vi "Ramping drive.vi"() -> ()   [LabVIEW 2017]
uses:
  <vilib>/Rock Robotics/WPI/ThirdParty/Phoenix-LabVIEW/Motor Controller/Controls/CTRE_Phoenix_MotorControl_ControlMode.ctl
  <vilib>/Rock Robotics/WPI/ThirdParty/Phoenix-LabVIEW/Motor Controller/Get/CTRE_Phoenix_MotorController_GetQuadratureData.vi
panel:
  in  "Max Speed/100Ms":dbl=650.0
  out "Acceleration Distance":dbl=8125.0
  in  "Ramp Seconds to full":dbl=2.5
  in  "Distance to Drive":dbl=5000.0
  in  "Distance tolerances":dbl=200.0
  out "TIMEOUTed":bool
  in  "TIMEOUT(S)":dbl=8.0
  # "NEED TALON DRIVE TO WORK"
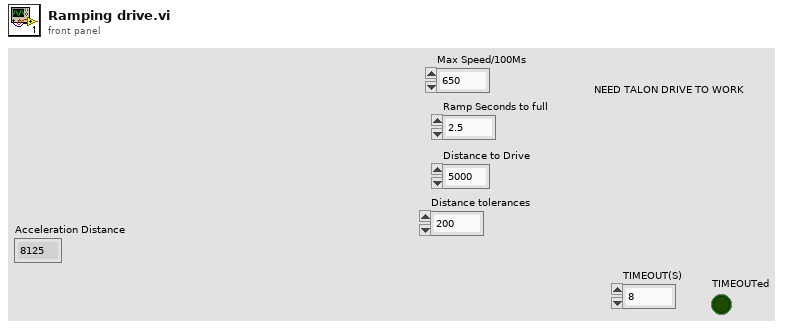
[diagram p1: front panel]
types:
  T1 = typedef "WPI_MotorControlDeviceRef.ctl" = cluster{"DeviceStatus":errorcluster, "Type":T2, "PWM":cluster{"PWM Channel":T3, "DeadBand":T4}, "CAN":cluster{"Device Number":u8, "SetOutput VI Ref":variant, "GetOutput VI Ref":variant, "Enable VI Ref":variant, "Disable VI Ref":variant, "Data":variant}, "Invert":bool, "DIO PWM":cluster{"PWM \"Enable\" Channel":T3, "DIOChannel":T5, "PWM Rate":dbl}}
  T2 = typedef "WPI_MotorControlType.ctl" = enum16{"PWM", "CAN", "DIO PWM"}
  T3 = typedef "FPGA_DIOPWMChannel.ctl" = enum8{"PWM 0", "PWM 1", "PWM 2", "PWM 3", "PWM 4", "PWM 5", "PWM 6", "PWM 7", "PWM 8", "PWM 9", "PWM MXP 0", "PWM MXP 1", "PWM MXP 2", "PWM MXP 3", "PWM MXP 4", "PWM MXP 5", "PWM MXP 6", "PWM MXP 7", "PWM MXP 8", "PWM MXP 9", "Invalid"}
  T4 = typedef "WPI_PWMDeadband.ctl" = cluster{"Name":string, "maxPositivePwm":i32, "minPositivePwm":i32, "centerPwm":i32, "maxNegativePwm":i32, "minNegativePwm":i32, "angularRange":u16}
  T5 = typedef "FPGA_DIOChannel.ctl" = enum8{"DIO 0", "DIO 1", "DIO 2", "DIO 3", "DIO 4", "DIO 5", "DIO 6", "DIO 7", "DIO 8", "DIO 9", "DIO MXP 0", "DIO MXP 1", "DIO MXP 2", "DIO MXP 3", "DIO MXP 4", "DIO MXP 5", "DIO MXP 6", "DIO MXP 7", "DIO MXP 8", "DIO MXP 9", "DIO MXP 10", "DIO MXP 11", "DIO MXP 12", "DIO MXP 13", "DIO MXP 14", "DIO MXP 15", "SPI Port CS1", "SPI Port CS2", "SPI Port CS3", "SPI Port MISO", "SPI Port MOSI", "Invalid"}
  T6 = typedef "CTRE_Phoenix_MotorControl_ControlMode.ctl" = u16
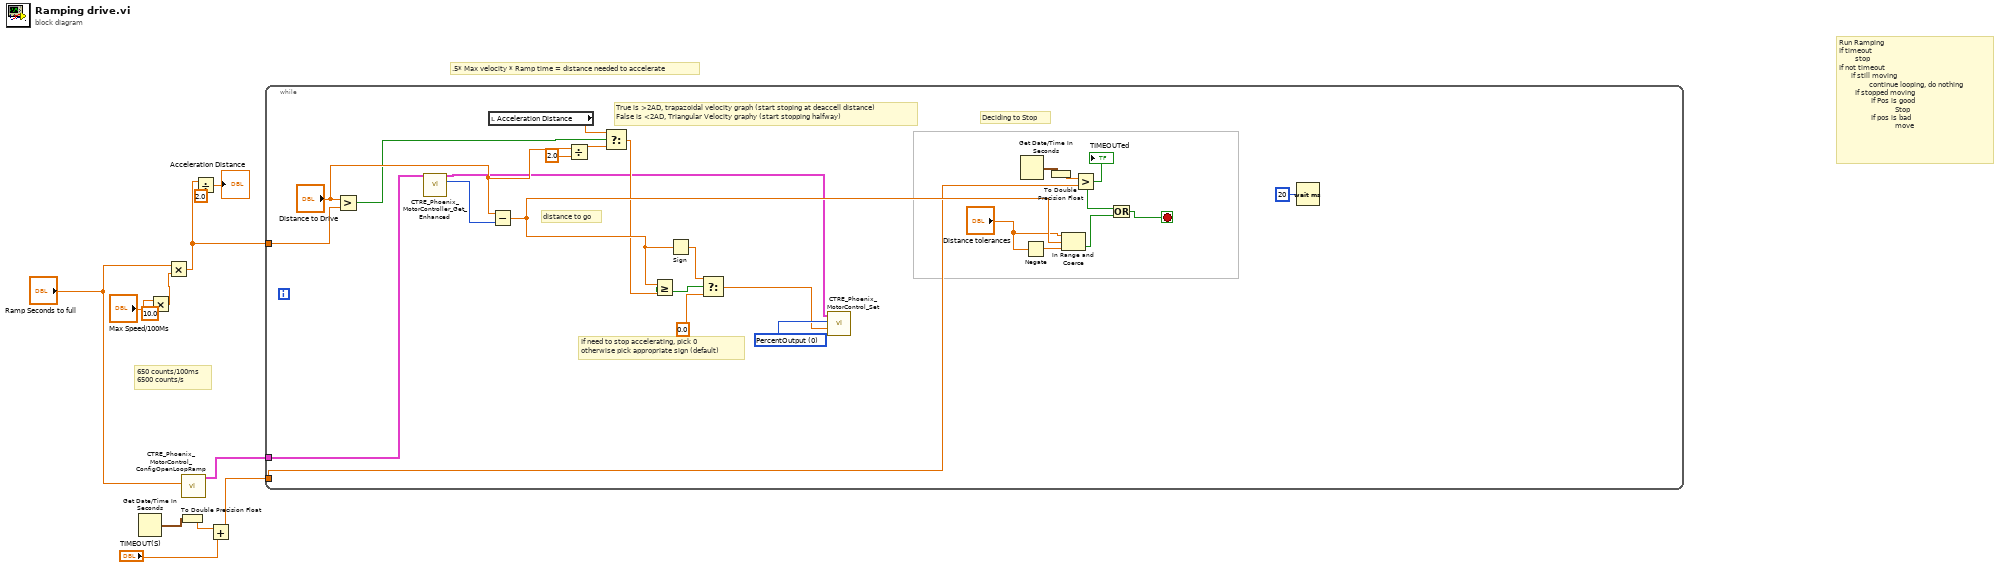
[diagram p0: block diagram]
diagram:
  # "Run Ramping\nIf timeout\n        stop\nIf not timeout\n      if still moving\n               continue looping, do nothing\n        If stopped moving\n                If Pos is good\n                            Stop\n                If pos is bad\n                            move"
  # ".5* Max velocity * Ramp time = distance needed to accelerate"
  # "650 counts/100ms\n6500 counts/s"
  n1 = Get Date/Time In Seconds() -> (seconds since 1Jan1904=w3:timestamp)
  n2 = Multiply(x="Max Speed/100Ms", y=10.0) -> (x*y=w6:dbl)
  n3 = Multiply(x="Ramp Seconds to full", y=w6) -> (x*y=w1:dbl)
  n4 = To Double Precision Float(number=w3) -> (double precision float=w2:dbl)
  n5 = call <vilib>:"CTRE_Phoenix_MotorControl_ConfigOpenLoopRamp.vi"("secondsFromNeutralToFull"="Ramp Seconds to full") -> (3:"PhoenixMotorControlDevRef"=w10:T1, 11:"PhoenixMotorControlDevRef"=w9:T1)  [unwired: 8 in, 1 out]
  n6 = Divide(x=w1, y=2.0) -> (x/y=→"Acceleration Distance":dbl)
  n7 = Add(x=w2, y="TIMEOUT(S)") -> (x+y=w4:dbl)
  n8 = while {
    tunnel: w10 -> [w39]
    tunnel: w4 -> [w36]
    tunnel: w1 -> [w34]
    stop <- w15 stop-if-true
    w26 = T6 0 items=["PercentOutput"=0, "Position"=1, "Velocity"=2, "Current"=3, "Follower"=5, "MotionProfile"=6, "MotionMagic"=7, "MotionMagicArc"=8, "MotionProfileArc"=10, "Disabled"=15] ("Control Mode")
    # "Deciding to Stop"
    # "If need to stop accelerating, pick 0\notherwise pick appropriate sign (default)"
    # "distance to go"
    # "True is >2AD, trapazoidal velocity graph (start stoping at deaccell distance)\nFalse is <2AD, Triangular Velocity graphy (start stopping halfway)"
    n9 = Greater?(x="Distance to Drive", y=w34) -> (0:w33:bool)
    n10 = call-poly <vilib>:"CTRE_Phoenix_MotorController_Get_Enhanced.vi"("PhoenixMotorControlDevRef"=w39) -> ("PhoenixMotorControlDevRef"=w14:T1, "Quadrature Position"=w23:i32)  [unwired: 11 in, 2 out]
    n11 = local read "Acceleration Distance"() -> (w29:dbl)
    n12 = Subtract(x="Distance to Drive", y=w23) -> (x-y=w38:dbl)
    n13 = Divide(x="Distance to Drive", y=2.0) -> (x/y=w28:dbl)
    n14 = Select(t=w29, s=w33, f=w28) -> (s? t:f=w22:dbl)
    n15 = Greater Or Equal?(x=w38, y=w22) -> (x >= y?=w24:bool)
    n16 = Sign(1:w38) -> (0:w32:dbl)
    n17 = Select(t=w32, s=w24, f=0.0) -> (s? t:f=w25:dbl)
    n18 = call <vilib>:"CTRE_Phoenix_MotorControl_Set.vi"("Output"=w25, "Control Mode"=w26, "PhoenixMotorControlDevRef"=w14) -> ("PhoenixMotorControlDevRef"=w37:T1)  [unwired: 7 in, 1 out]
    n19 = Get Date/Time In Seconds() -> (seconds since 1Jan1904=w19:timestamp)
    n20 = Negate(x="Distance tolerances") -> (-x=w20:dbl)
    n21 = To Double Precision Float(number=w19) -> (double precision float=w18:dbl)
    n22 = In Range and Coerce(upper limit="Distance tolerances", x=w38, lower limit=w20) -> (In Range?=w16:bool)  [unwired: 1 out]
    n23 = Greater?(x=w18, y=w36) -> (0:w17:bool)
    "TIMEOUTed" <- w17
    n24 = Or(x=w17, y=w16) -> (x .or. y?=w15:bool)
    n25 = Wait (ms)(milliseconds to wait=u32 20) -> ()  [unwired: 1 out]
  }
